vi "String_Tokenize.vi"(1 "String Token":string, 2 "String":string) -> (0 "String Array":string[](array[string]))   [LabVIEW 2018]
doc: "Split a string with elements separated by known token into an array of substrings\n\nR. Sheehan 10 - 8 - 2018"
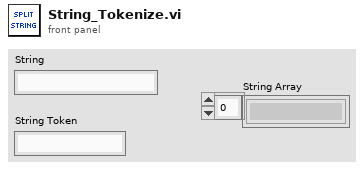
[diagram p1: front panel]
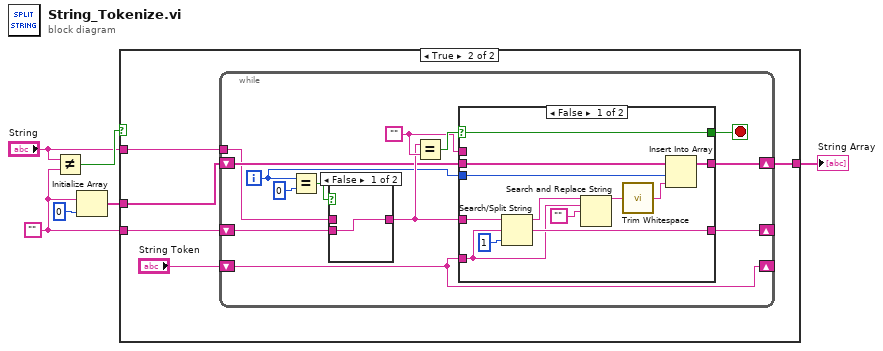
[diagram p0: block diagram]
diagram:
  w5 = ""
  n1 = Not Equal?(x="String", y=w5) -> (x != y?=w3:bool)
  n2 = Initialize Array(w5, 0 ("dimension size")) -> (w4:string[])
  n3 = case shown="True" w3 {
    tunnel: w5 -> [_ w12]
    tunnel: w4 -> [w7 w11]
    tunnel: "String" -> [_ w9]
    tunnel: [w7 w10] -> w1
    frame False {
    }
    frame True {
      n4 = while {
        shift-right: [w18] -> _
        shift-left: w12 -> [w20]
        shift-right: [w15] -> w10
        shift-left: w11 -> [w17]
        tunnel: w9 -> [w14]
        shift-right: [w13] -> _
        shift-left: "String Token" -> [w13]
        i -> [w16]
        stop <- w24 stop-if-true
        w23 = ""
        n5 = Equal?(x=w16, y=0) -> (x = y?=w21:bool)
        n6 = case shown="False" w21 {
          tunnel: [w26 w27] -> w19
          tunnel: w20 -> [w26 _]
          tunnel: w14 -> [_ w27]
          frame False {
          }
          frame True {
          }
        }
        n7 = Equal?(x=w19, y=w23) -> (x = y?=w25:bool)
        n8 = case shown="False" w25 {
          selector: w25 -> [w39 w42]
          tunnel: [w39 w42] -> w24
          tunnel: [w37 w41] -> w18
          tunnel: w23 -> [_ w41]
          tunnel: w19 -> [w38 _]
          tunnel: w17 -> [w32 w40]
          tunnel: w16 -> [w36 _]
          tunnel: [w31 w40] -> w15
          tunnel: w13 -> [w28 _]
          frame False {
            n9 = Search/Split String(string=w38, search string/char (-)=w28, offset (0)=1) -> (substring before match=w34:string, match + rest of string=w37:string)  [unwired: 1 out]
            n10 = Search and Replace String(input string=w34, search string=w28, replace string="") -> (result string=w33:string)  [unwired: 5 in, 3 out]
            n11 = call <vilib>:"Trim Whitespace.vi"("string"=w33) -> ("trimmed string"=w30:string)  [unwired: 1 in]
            n12 = Insert Into Array(array=w32, index=w36, new element=w30) -> (w31:string[])
          }
          frame True {
          }
        }
      }
    }
  }
  "String Array" <- w1
